vi "WPI_UtilitiesDiscover Robot.vi"(11 "Team Number":string) -> (2 "Team Robots":string[](array[string]), 3 "Static IP":u32 format="%x")   [LabVIEW 2017]
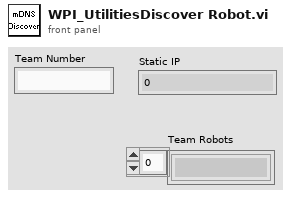
[diagram p1: front panel]
types:
  T1 = typedef "mdnsResolveInstance.ctl" = cluster{"name":string, "macAddress":string, "hostname":string, "ipAddress":string, "productId":string, "serialNumber":string, "systemStatus":string, "ifIndex":u32}
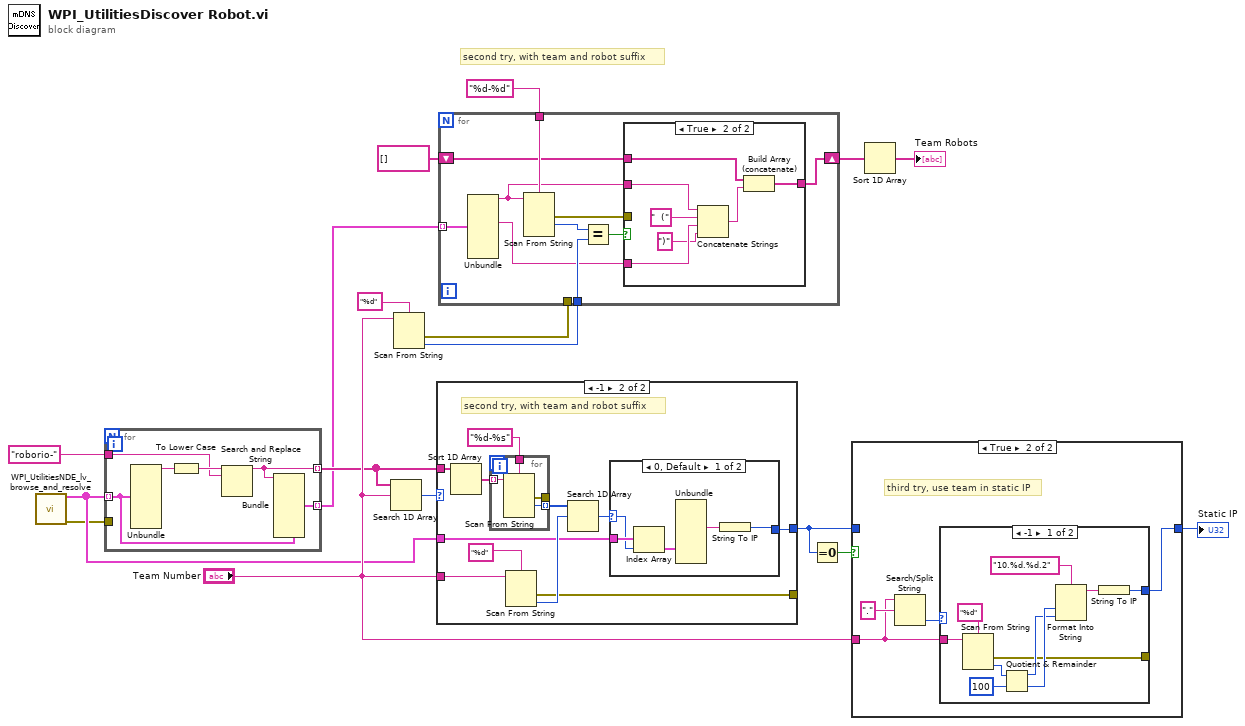
[diagram p0: block diagram]
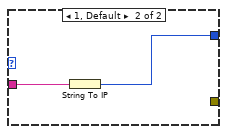
[diagram p4: hidden frame]
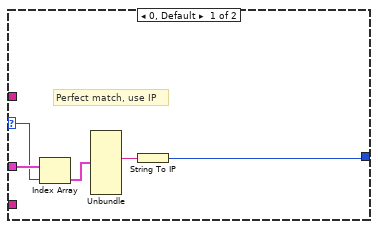
[diagram p5: hidden frame]
diagram:
  # "second try, with team and robot suffix"
  n1 = call <vilib>:"WPI_UtilitiesNDE_lv_browse_and_resolve.vi"() -> ("instances"=w7:T1[], "error out"=w1:errorcluster)  [unwired: 14 in]
  n2 = for {
    tunnel: w7 -> [w20] mode=indexing
    tunnel: "roborio-" ("format string") -> [w21]
    tunnel: [w19] -> w6 mode=indexing
    tunnel: [w18] -> w5 mode=indexing
    tunnel: w1 -> [_]
    n3 = Unbundle(w20) -> ("name"=w23:string)  [unwired: 7 out]
    n4 = To Lower Case(string=w23) -> (all lower case string=w22:string)
    n5 = Search and Replace String(input string=w22, search string=w21) -> (result string=w19:string)  [unwired: 6 in, 3 out]
    n6 = Bundle(cluster=w20, "name"=w19) -> (w18:T1)  [unwired: 7 in]
  }
  n7 = Search 1D Array(1D array=w6, element="Team Number") -> (index of element=w17:i32)  [unwired: 1 in]
  n8 = Scan From String(format string="%d", input string="Team Number") -> (error out=w8:errorcluster, output 1=w9:i32)  [unwired: 3 in, 2 out]
  n9 = case shown="-1" w17 {
    selector: w17 -> [w27 _]
    tunnel: w7 -> [w28 w33]
    tunnel: w6 -> [_ w32]
    tunnel: "Team Number" -> [_ w38]
    tunnel: [w24 w30] -> w13
    tunnel: [_ w29] -> _
    frame 0, Default {
      # "Perfect match, use IP"
      n10 = Index Array(array=w28, index=w27) -> (element=w25:T1)
      n11 = Unbundle(w25) -> ("ipAddress"=w26:string)  [unwired: 7 out]
      n12 = String To IP(1:w26) -> (0:w24:u32)
    }
    frame -1 {
      # "second try, with team and robot suffix"
      n13 = Sort 1D Array(array=w32) -> (sorted array=w31:string[])
      n14 = for {
        tunnel: w31 -> [w48] mode=indexing
        tunnel: "%d-%s" ("format string") -> [w47]
        tunnel: [w46] -> w36 mode=indexing
        tunnel: [w45] -> _
        n15 = Scan From String(format string=w47, input string=w48) -> (error out=w45:errorcluster, output 1=w46:i32)  [unwired: 5 in, 2 out]
      }
      n16 = Scan From String(format string="%d", input string=w38) -> (error out=w29:errorcluster, output 1=w35:i32)  [unwired: 3 in, 2 out]
      n17 = Search 1D Array(1D array=w36, element=w35) -> (index of element=w34:i32)  [unwired: 1 in]
      n18 = case shown="0, Default" w34 {
        selector: w34 -> [w43 _]
        tunnel: w33 -> [w44 _]
        tunnel: [w40 _] -> w30
        frame 0, Default {
          n19 = Index Array(array=w44, index=w43) -> (element=w42:T1)
          n20 = Unbundle(w42) -> ("ipAddress"=w41:string)  [unwired: 7 out]
          n21 = String To IP(1:w41) -> (0:w40:u32)
        }
        frame -1 {
        }
      }
    }
  }
  n22 = for {
    tunnel: "%d-%d" ("format string") -> [w58]
    tunnel: w9 -> [w56]
    tunnel: w8 -> [_]
    tunnel: w5 -> [w53] mode=indexing
    shift-right: [w49] -> w3
    shift-left: string[] [] -> [w50]
    n23 = Unbundle(w53) -> ("name"=w51:string, "ipAddress"=w52:string)  [unwired: 6 out]
    n24 = Scan From String(format string=w58, input string=w51) -> (error out=w54:errorcluster, output 1=w57:i32)  [unwired: 5 in, 2 out]
    n25 = Equal?(x=w57, y=w56) -> (x = y?=w55:bool)
    n26 = case shown="True" w55 {
      tunnel: w54 -> [_ _]
      tunnel: w52 -> [_ w64]
      tunnel: w51 -> [_ w66]
      tunnel: w50 -> [w59 w62]
      tunnel: [w59 w61] -> w49
      frame False {
      }
      frame True {
        n27 = Concatenate Strings(w66, "  (" ("format string"), w64, ")" ("format string")) -> (w63:string)
        n28 = Build Array (concatenate)(w62, w63) -> (w61:string[])
      }
    }
  }
  n29 = Equal To 0?(x=w13) -> (x = 0?=w15:bool)
  n30 = case shown="True" w15 {
    tunnel: "Team Number" -> [_ w69]
    tunnel: [w67 w68] -> w14
    tunnel: w13 -> [w67 _]
    frame False {
    }
    frame True {
      # "third try, use team in static IP"
      n31 = Search/Split String(string=w69, search string/char (-)=".") -> (offset of match=w70:i32)  [unwired: 1 in, 2 out]
      n32 = case shown="-1" w70 {
        tunnel: w69 -> [w80 w83]
        tunnel: [w73 w82] -> w68
        tunnel: [w72 _] -> _
        frame -1 {
          n33 = Scan From String(format string="%d", input string=w80) -> (error out=w72:errorcluster, output 1=w77:i32)  [unwired: 3 in, 2 out]
          n34 = Quotient & Remainder(x=w77, y=i16 100 ("width (-)")) -> (x-y*floor(x/y)=w75:i32, floor(x/y)=w76:i32)
          n35 = Format Into String(format string="10.%d.%d.2", w76, w75) -> (resulting string=w74:string)  [unwired: 2 in, 1 out]
          n36 = String To IP(1:w74) -> (0:w73:u32)
        }
        frame 1, Default {
          n37 = String To IP(1:w83) -> (0:w82:u32)
        }
      }
    }
  }
  "Static IP" <- w14
  n38 = Sort 1D Array(array=w3) -> (sorted array=→"Team Robots":string[])
